vi "Coverage Analyzer View.vi"(8 "error in (no error)":errorcluster, 11 "Coverage Analyzer Result View.lvclass":refnum<class "Coverage Analyzer Result View.lvclass">) -> (0 "error out":errorcluster)   [LabVIEW 2020, in "Coverage Analyzer Result View.lvclass"]
uses:
  Coverage Analyzer Result View.lvclass
  Coverage Analyzer Result View.lvclass/Coverage Analyzer Result View.ctl
panel:
  in  "Method Test Times":i32(listbox)
  out "Coverage for Executed VIs":string
  out "Fraction of VIs Executed":string
  in  "Hide VIs not executed?":bool=TRUE
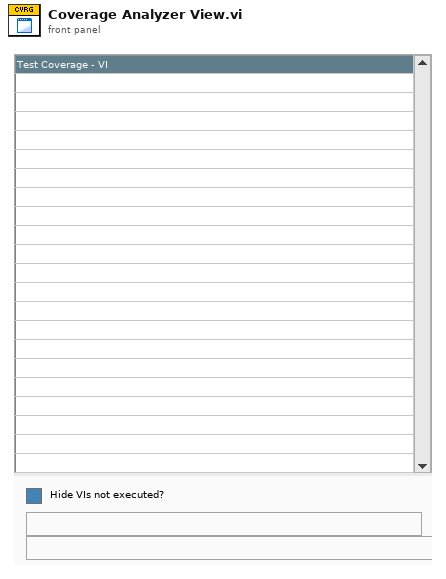
[diagram p1: front panel]
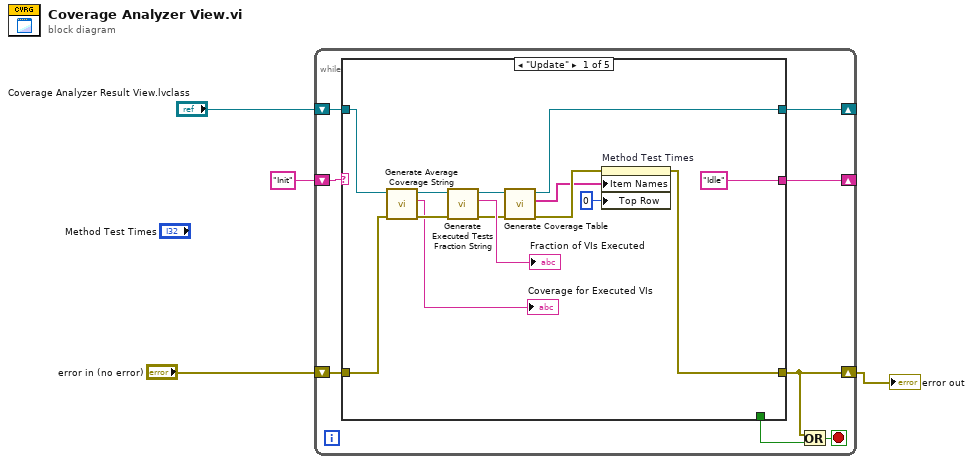
[diagram p0: block diagram]
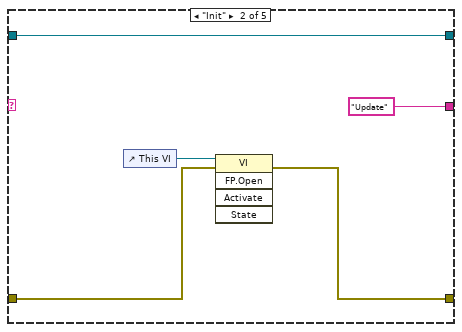
[diagram p2: hidden frame]
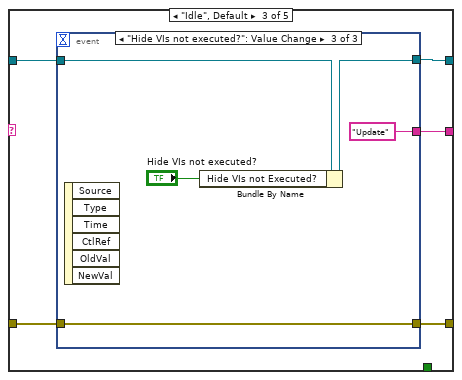
[diagram p3: hidden frame]
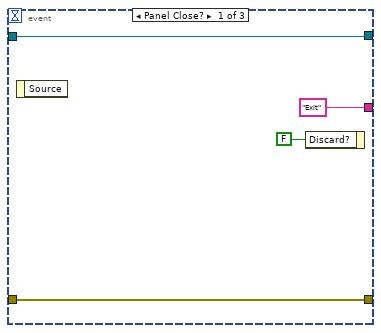
[diagram p4: hidden frame]
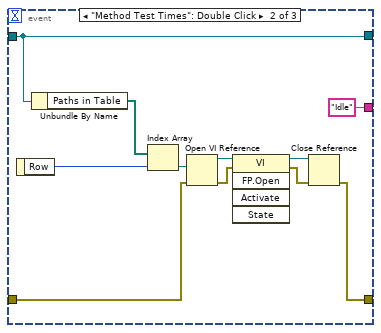
[diagram p5: hidden frame]
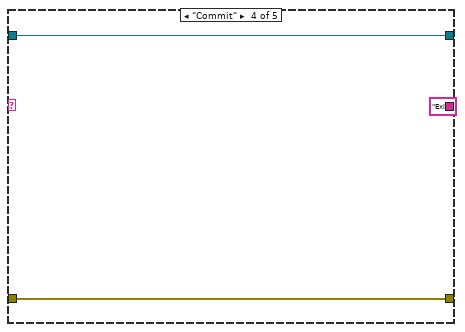
[diagram p6: hidden frame]
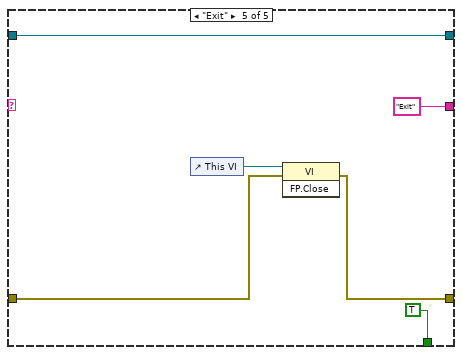
[diagram p7: hidden frame]
diagram:
  n1 = while {
    shift-right: [w9] -> _
    shift-left: "Coverage Analyzer Result View.lvclass" -> [w10]
    shift-right: [w5] -> w2
    shift-left: "error in (no error)" -> [w11]
    shift-right: [w8] -> _
    shift-left: "Init" -> [w12]
    stop <- w6 stop-if-true
    n2 = case shown="\"Update\"" w12 {
      tunnel: [w25 w29 w36 w59 w61] -> w5
      tunnel: w11 -> [w19 w28 w35 w59 w60]
      tunnel: w10 -> [w16 w27 w34 w58 w65]
      tunnel: [w22 w27 w33 w58 w65] -> w9
      tunnel: ["Idle" "Update" w32 "Exit" "Exit"] -> w8
      tunnel: [_ _ _ _ TRUE] -> w7
      frame "Update" {
        n3 = call "Generate Average Coverage String.vi"("error in (no error)"=w19, "Coverage Analyzer Result View in"=w16) -> ("error out"=w17:errorcluster, "Fraction of VIs Executed"=→"Coverage for Executed VIs":string, "Coverage Analyzer Result View out"=w15:refnum<class "Coverage Analyzer Result View.lvclass">)  [unwired: 7 in]
        n4 = call "Generate Executed Tests Fraction String.vi"("error in (no error)"=w17, "Coverage Analyzer Result View in"=w15) -> ("error out"=w18:errorcluster, "Fraction of VIs Executed"=→"Fraction of VIs Executed":string, "Coverage Analyzer Result View out"=w20:refnum<class "Coverage Analyzer Result View.lvclass">)  [unwired: 7 in]
        n5 = call "Generate Coverage Table.vi"("error in (no error)"=w18, "Coverage Analyzer Result View In"=w20) -> ("error out"=w24:errorcluster, "Item Names"=w23:string[], "Coverage Analyzer Result View Out"=w22:refnum<class "Coverage Analyzer Result View.lvclass">)  [unwired: 7 in]
        n6 = property on="Method Test Times" class="LstBox (strict)"(error in=w24, "Item Names"=w23, "Top Row"=0) -> (error out=w25:errorcluster)  [unwired: 1 in, 1 out]
      }
      frame "Init" {
        n7 = control-ref of="This VI"() -> (w30:refnum<vi>)
        n8 = invoke class="VI" method="FP.Open"(reference=w30, error in=w28) -> (error out=w29:errorcluster)  [unwired: 3 in, 4 out]
      }
      frame "Idle", Default {
        n9 = event shown="[2] \"Hide VIs not executed?\": Value Change" {
          selector: _ -> [_ _ _]
          dyn-events: _ -> [_ _ _]
          timeout: _ -> [_ _ _]
          tunnel: [w40 w42 w56] -> w36
          tunnel: w35 -> [w40 w41 w56]
          tunnel: w34 -> [w39 w50 w55]
          tunnel: [w39 w50 w53] -> w33
          tunnel: ["Exit" "Idle" "Update"] -> w32
          event Panel Close? {
            n10 = event-data() -> ()  [unwired: 1 in, 1 out]
            n11 = event-data("Discard?"=FALSE) -> ()  [unwired: 1 in, 1 out]
          }
          event "Method Test Times": Double Click {
            n12 = event-data() -> ("Row"=w48:i32)  [unwired: 1 in]
            n13 = Unbundle By Name(w50) -> ("Paths in Table"=w49:path[])
            n14 = Index Array(array=w49, index=w48) -> (element=w47:path)
            n15 = Open VI Reference(vi path=w47, error in (no error)=w41) -> (vi reference=w46:refnum<vi>, error out=w45:errorcluster)  [unwired: 4 in]
            n16 = invoke class="VI" method="FP.Open"(reference=w46, error in=w45) -> (reference out=w44:refnum<vi>, error out=w43:errorcluster)  [unwired: 3 in, 3 out]
            n17 = Close Reference(reference=w44, error in (no error)=w43) -> (error out=w42:errorcluster)
          }
          event "Hide VIs not executed?": Value Change {
            n18 = event-data() -> ()  [unwired: 1 in, 6 out]
            n19 = Bundle By Name(cluster=w55, "Hide VIs not Executed?"="Hide VIs not executed?") -> (w53:refnum<class "Coverage Analyzer Result View.lvclass">)
          }
        }
      }
      frame "Commit" {
      }
      frame "Exit" {
        n20 = control-ref of="This VI"() -> (w62:refnum<vi>)
        n21 = invoke class="VI" method="FP.Close"(reference=w62, error in=w60) -> (error out=w61:errorcluster)  [unwired: 1 in, 2 out]
      }
    }
    n22 = Or(x=w5, y=w7) -> (x .or. y?=w6:bool)
  }
  "error out" <- w2
